vi "Main.vi"() -> ()   [LabVIEW 2017]
uses:
  Subvi/Baidu api/Baidu api.lvlib
  <vilib>/httpClient/LabVIEWHTTPClient.lvlib
  Subvi/Encode Base64/Encode Base64.lvlib
panel:
  in  "人脸检测":bool
  out "Image Display":T1(plugin-control)
  in  "face_fields":T2
  out "body":string caption="体部"
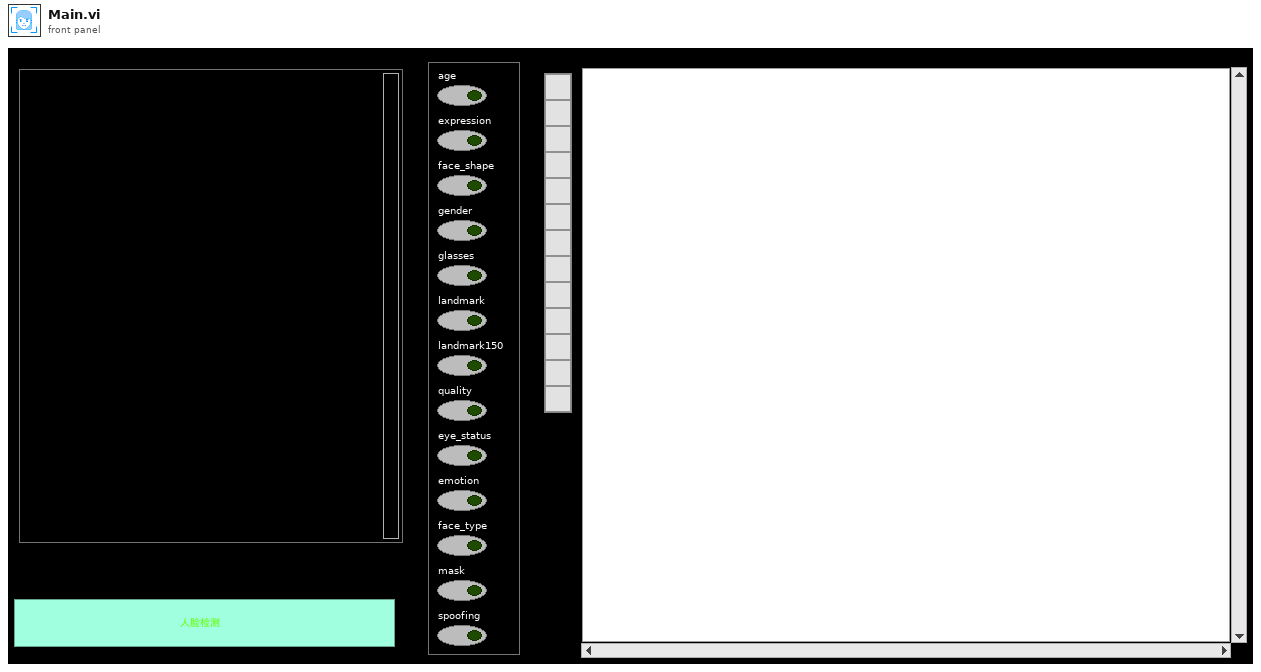
[diagram p1: front panel]
types:
  T1 = typedef "IMAQ Image.ctl" = refnum<image>
  T2 = cluster{"age":bool, "expression":bool, "face_shape":bool, "gender":bool, "glasses":bool, "landmark":bool, "landmark150":bool, "quality":bool, "eye_status":bool, "emotion":bool, "face_type":bool, "mask":bool, "spoofing":bool}
  T3 = typedef "Image Type" = u32
  T4 = typedef "LabVIEWHTTPClient.lvlib/ClientHandle.ctl" = refnum<k1>
  T5 = cluster{"image":string, "image_type":string, "face_fields ":cluster{"age":bool, "expression":bool, "face_shape":bool, "gender":bool, "glasses":bool, "landmark":bool, "landmark150":bool, "quality":bool, "eye_status":bool, "emotion":bool, "face_type":bool, "mask":bool, "spoofing":bool}}
  T6 = typedef "face_list.ctl" = cluster{"location":cluster{"left":i32, "top":i32, "width":i32, "height":i32, "Rotation":i32}, "face_probability":dbl, "age":dbl, "landmark":cluster{"x":u32, "y":u32}[], "landmark72":cluster{"x":u32, "y":u32}[], "angle":cluster{"yaw":dbl, "pitch":dbl, "roll":dbl}, "face_token":string, "face_shape":cluster{"type":string, "probability":dbl}, "glasses":cluster{"type":string, "probability":dbl}, "expression":cluster{"type":string, "probability":dbl}, "gender":cluster{"type":string, "probability":dbl}, "quality":cluster{"illumination":i32, "completeness":i32, "blur":i32, "occlusion":cluster{"left_eye":dbl, "right_eye":dbl, "nose":dbl, "mouth":dbl, "left_cheek":dbl, "right_cheek":dbl, "chin":dbl}}}
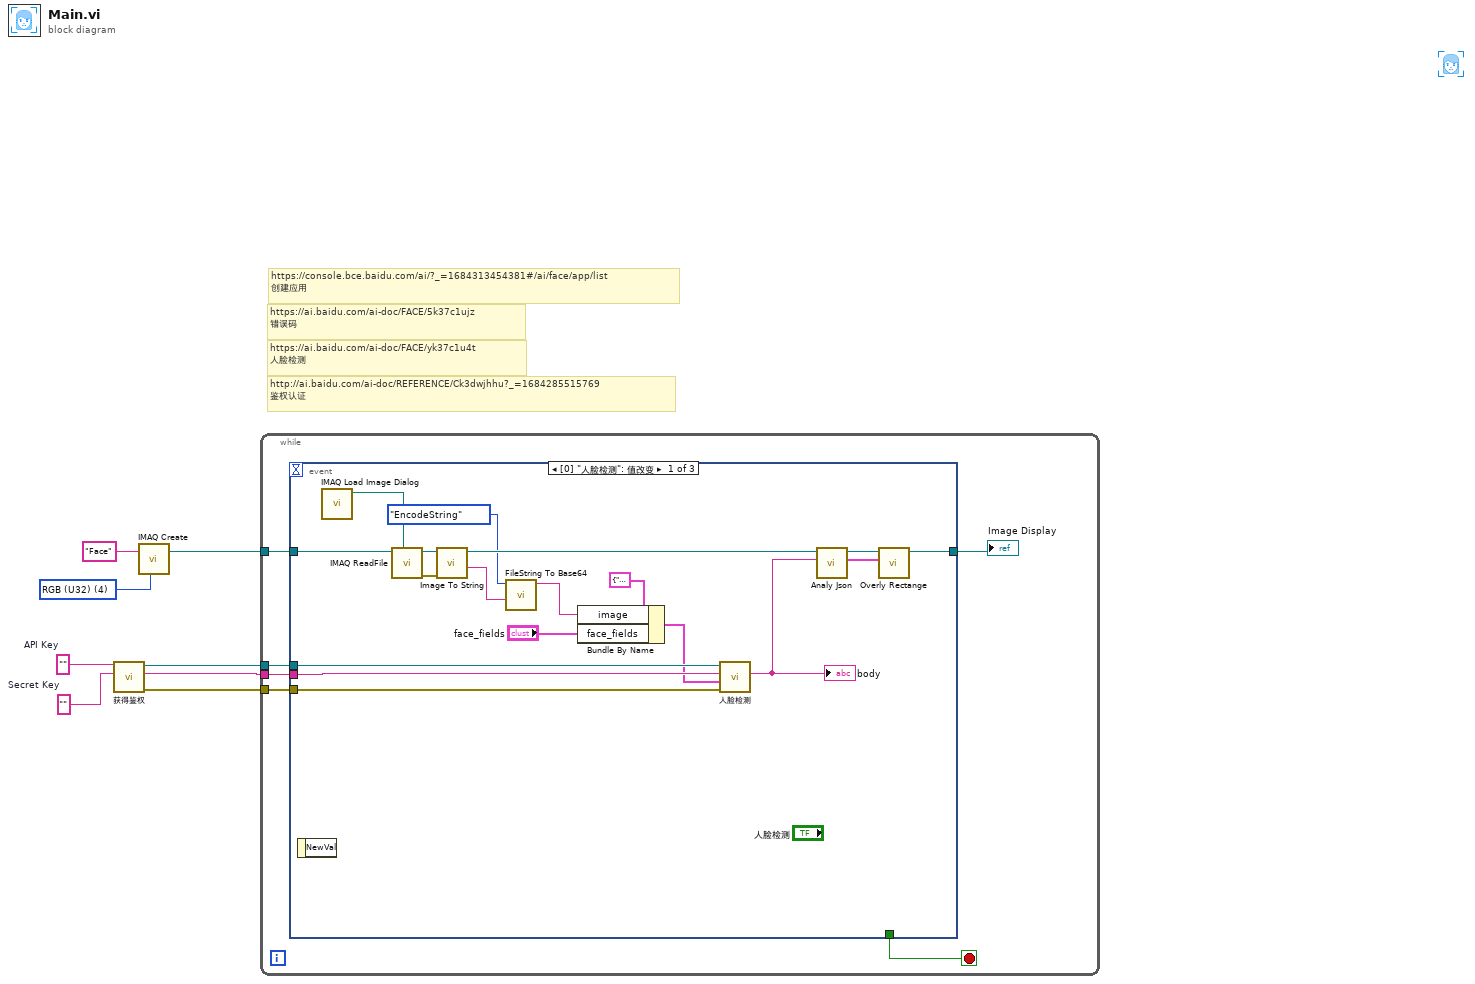
[diagram p0: block diagram]
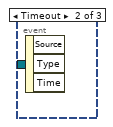
[diagram p2: hidden frame]
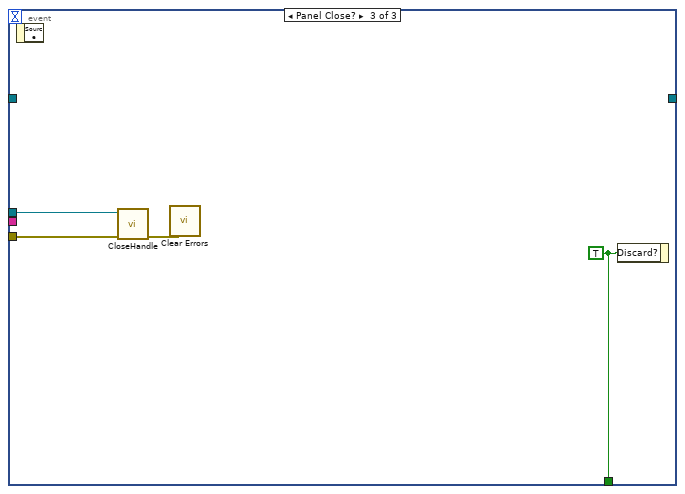
[diagram p3: hidden frame]
diagram:
  w4 = T3 4 items=["Grayscale (U8)", "Grayscale (I16)", "Grayscale (SGL)", "Complex (CSG)", "RGB (U32)", "HSL (U32)", "RGB (U64)", "Grayscale (U16)"] ("Image Type")
  w8 = ""  # Secret Key
  w7 = ""  # API Key
  # "https://console.bce.baidu.com/ai/?_=1684313454381#/ai/face/app/list\n创建应用"
  # "http://ai.baidu.com/ai-doc/REFERENCE/Ck3dwjhhu?_=1684285515769\n鉴权认证"
  # "https://ai.baidu.com/ai-doc/FACE/yk37c1u4t\n人脸检测"
  # "https://ai.baidu.com/ai-doc/FACE/5k37c1ujz\n错误码"
  n1 = call "获得鉴权.vi"("Secret Key"=w8, "API Key"=w7) -> ("错误输出"=w5:errorcluster, "access_token"=w2:string, "client handle out"=w6:T4)  [unwired: 7 in]
  n2 = call "IMAQ Create"("Image Name"="Face", "Image Type"=w4) -> ("New Image"=w3:T1)  [unwired: 3 in, 1 out]
  n3 = while {
    tunnel: w6 -> [w13]
    tunnel: w5 -> [w12]
    tunnel: w3 -> [w11]
    tunnel: w2 -> [w10]
    stop <- w14 stop-if-true
    n4 = event shown="[0] \"人脸检测\": 值改变" {
      selector: _ -> [_ _ _]
      dyn-events: _ -> [_ _ _]
      timeout: _ -> [_ _ _]
      tunnel: [_ _ w35] -> w14
      tunnel: w13 -> [w30 _ w34]
      tunnel: w12 -> [w28 _ w33]
      tunnel: w11 -> [w21 _ _]
      tunnel: w10 -> [w29 _ _]
      tunnel: [w26 _ _] -> w9
      event "人脸检测": Value Change {
        n5 = event-data() -> ()  [unwired: 1 in, 1 out]
        n6 = call "IMAQ Load Image Dialog"() -> ("Path"=w31:path)  [unwired: 9 in, 2 out]
        n7 = call "IMAQ ReadFile"("File Path"=w31, "Image"=w21) -> ("error out"=w18:errorcluster, "Image Out"=w20:T1)  [unwired: 5 in, 3 out]
        n8 = call "Image To String.vi"("错误输入（无错误）"=w18, "引用句柄输入"=w20) -> ("FileString"=w17:string, "引用句柄输出"=w19:T1)  [unwired: 6 in, 1 out]
        n9 = call "FileString To Base64.vi"("String"=w17, "Action"=enum16{"EncodeString", "EcodeFile"}."EncodeString") -> ("encodeURIComponent"=w15:string)  [unwired: 6 in, 3 out]
        n10 = Bundle By Name(cluster=T5 {"image"="", "image_type"="BASE64", "face_fields "={"age"=FALSE, "expression"=FALSE, "face_shape"=FALSE, "gender"=FALSE, "glasses"=FALSE, "landmark"=FALSE, "landmark150"=FALSE, "quality"=FALSE, "eye_status"=FALSE, "emotion"=FALSE, "face_type"=FALSE, "mask"=FALSE, "spoofing"=FALSE}} ("face Parameter"), "image"=w15, "face_fields"="face_fields") -> (w22:T5)
        n11 = call "人脸检测.vi"("错误输入（无错误）"=w28, "face Parameter"=w22, "access_token"=w29, "client_in"=w30) -> ("body"=w25:string)  [unwired: 5 in, 2 out]
        "body" <- w25
        n12 = call "Analy Json.vi"("body"=w25) -> ("face_list"=w27:T6[])  [unwired: 8 in, 2 out]
        n13 = call "Overly Rectange.vi"("face_list"=w27, "Image In"=w19) -> ("Image Out"=w26:T1)  [unwired: 8 in, 1 out]
      }
      event Timeout {
        n14 = event-data() -> ()  [unwired: 1 in, 3 out]
      }
      event Panel Close? {
        w35 = TRUE ("放弃？")
        n15 = event-data() -> ()  [unwired: 1 in, 1 out]
        n16 = call <vilib>:"CloseHandle.vi"("client handle"=w34, "error in (no error)"=w33) -> ("error out"=w32:errorcluster)  [unwired: 13 in]
        n17 = call <vilib>:"Clear Errors.vi"("error in (no error)"=w32) -> ()  [unwired: 5 in, 2 out]
        n18 = event-data("Discard?"=w35) -> ()  [unwired: 1 in, 1 out]
      }
    }
    "Image Display" <- w9
  }
